vi "Configure Notice Beeper.vi"(8 "error in (no error)":errorcluster, 10 "Enable Notice Beeper  (F: Disable)":bool, 11 "VISA resource name":refnum<visa-resource-name>) -> (0 "error out":errorcluster, 3 "VISA resource name out":refnum<visa-resource-name>)   [LabVIEW 2017, in "ADCMT 6240.lvlib"]
doc: "Configures the notice beeper setting."
uses:
  ADCMT 6240.lvlib
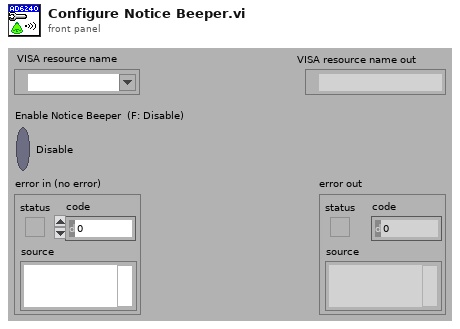
[diagram p1: front panel]
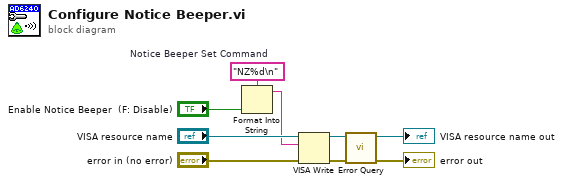
[diagram p0: block diagram]
diagram:
  w3 = "NZ%d\n"  # Notice Beeper Set Command
  n1 = Format Into String(format string=w3, "Enable Notice Beeper  (F: Disable)") -> (resulting string=w1:string)  [unwired: 2 in, 1 out]
  n2 = VISA Write ("VISA書き込み")(VISA resource name="VISA resource name", write buffer=w1, error in (no error)="error in (no error)") -> (VISA resource name out=w5:refnum<visa-resource-name>, error out=w4:errorcluster)  [unwired: 1 out]
  n3 = call "Error Query.vi"("error in (no error)"=w4, "VISA resource name"=w5) -> ("error out"=→"error out":errorcluster, "VISA resource name out"=→"VISA resource name out":refnum<visa-resource-name>)  [unwired: 6 in, 2 out]
